vi "FTW-JSON-Interpret-Array-String.vi"(1 "Escaped JSON Strings":string[](array[string])) -> (0 "LabVIEW Strings":string[](array[string]))   [LabVIEW 2012]
uses:
  FTW-JSON-RegexParse.vi
  Regex/FTW-Regex.vi
  FTW-JSON-RegexHeader.vi
  Error/FTW-ERR-ThrowError.vi
  FTW-JSON-Unescape.vi
panel:
  # "Inputs"
  # "Outputs"
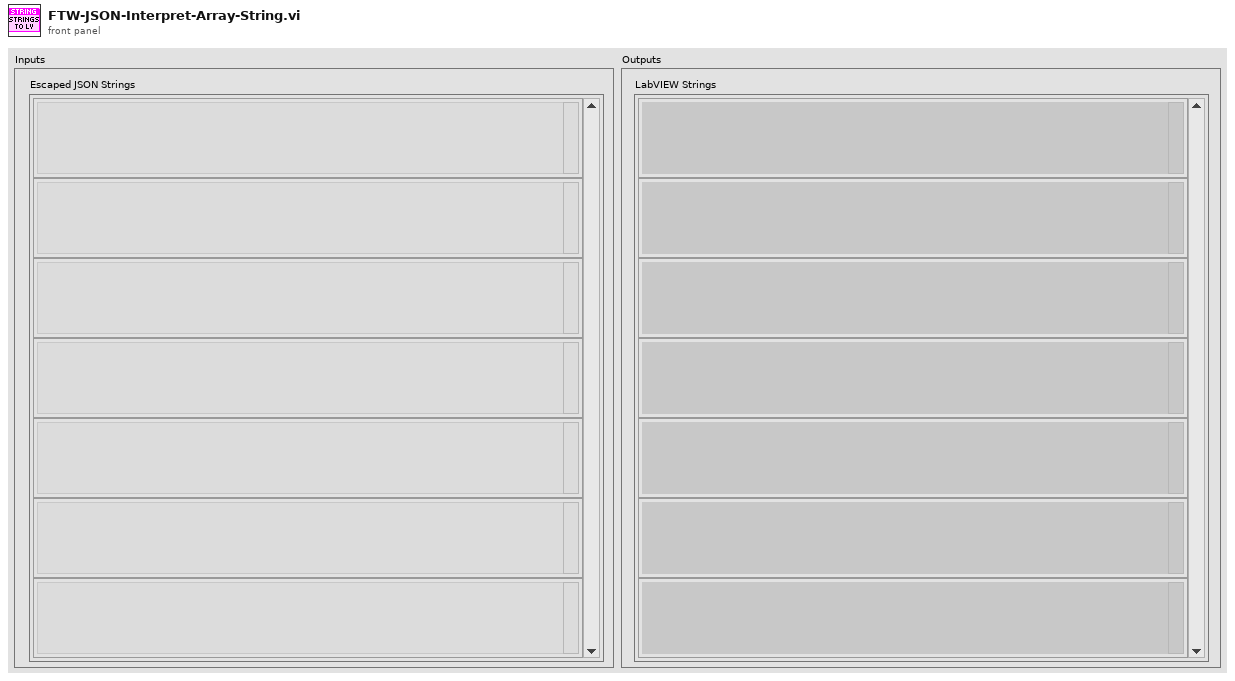
[diagram p1: front panel]
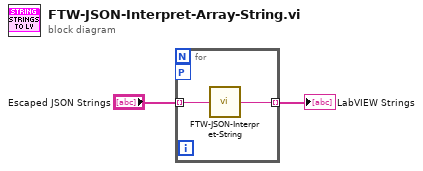
[diagram p0: block diagram]
diagram:
  n1 = for {
    tunnel: "Escaped JSON Strings" -> [w4] mode=indexing
    tunnel: [w3] -> w1 mode=indexing
    workers-P: _ -> [_]
    n2 = call "FTW-JSON-Interpret-String.vi"("JSON String"=w4) -> ("LabVIEW String"=w3:string)
  }
  "LabVIEW Strings" <- w1
